vi "处理-输入数值.vi"(8 "error in (no error)":errorcluster caption="错误输入（无错误）", 11 "计算器类 输入":refnum<class "计算器类.lvclass">) -> (0 "error out":errorcluster caption="错误输出", 3 "计算器类 输出":refnum<class "计算器类.lvclass">)   [LabVIEW 2020, in "计算器类.lvclass"]
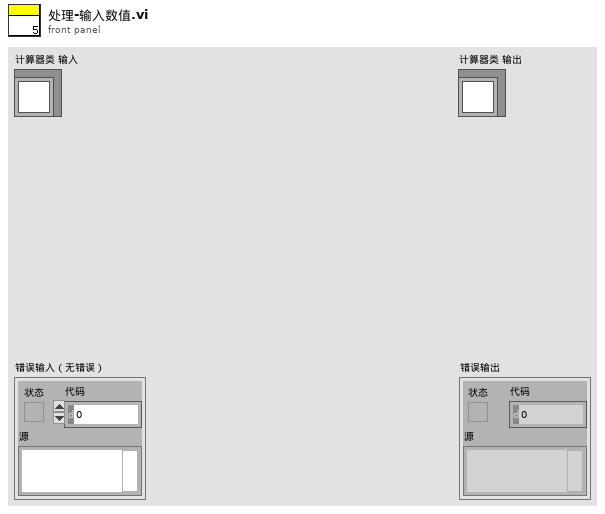
[diagram p1: front panel]
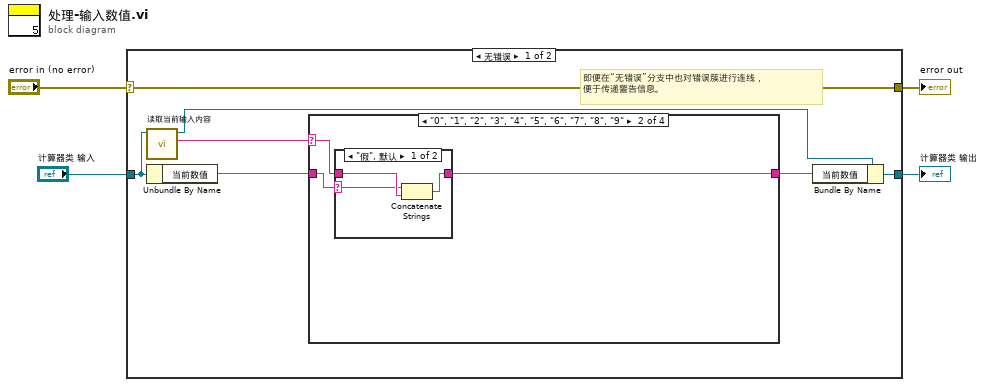
[diagram p0: block diagram]
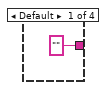
[diagram p2: hidden frame]
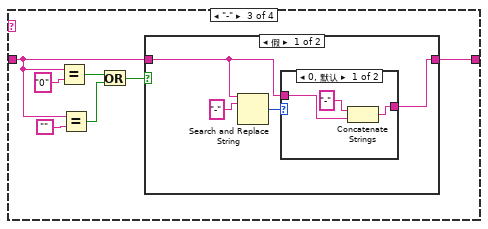
[diagram p4: hidden frame]
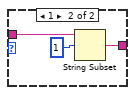
[diagram p5: hidden frame]
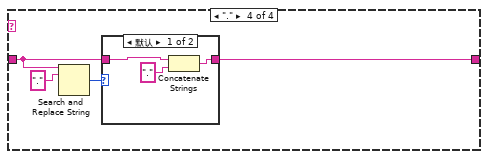
[diagram p7: hidden frame]
diagram:
  n1 = case shown="无错误" "error in (no error)" {
    selector: "error in (no error)" -> [w11 w47]
    tunnel: [w11 w47] -> w3
    tunnel: [w9 w46] -> w1
    tunnel: "计算器类 输入" -> [w6 w46]
    frame No Error {
      # "即便在“无错误”分支中也对错误簇进行连线，\n便于传递警告信息。"
      n2 = call "读取当前输入内容.vi"("计算器类输入"=w6) -> ("当前输入内容"=w7:string, "计算器类输出"=w5:refnum<class "计算器类.lvclass">)  [unwired: 8 in, 1 out]
      n3 = Unbundle By Name(w6) -> ("当前数值"=w10:string)
      n4 = case shown="\"0\", \"1\", \"2\", \"3\", \"4\", \"5\", \"6\", \"7\", \"8\", \"9\"" w7 {
        selector: w7 -> [_ w14 _ _]
        tunnel: w10 -> [_ w15 w21 w39]
        tunnel: ["" ("Value") w13 w20 w38] -> w8
        frame Default {
        }
        frame "0", "1", "2", "3", "4", "5", "6", "7", "8", "9" {
          n5 = case shown="\"假\", 默认" w15 {
            selector: w15 -> [w17 _]
            tunnel: w14 -> [w18 w19]
            tunnel: [w16 w19] -> w13
            frame "假", Default {
              n6 = Concatenate Strings(w17, w18) -> (w16:string)
            }
            frame "0" {
            }
          }
        }
        frame "-" {
          n7 = Equal?(x=w21, y="0") -> (x = y?=w24:bool)
          n8 = Equal?(x=w21, y="") -> (x = y?=w23:bool)
          n9 = Or(x=w24, y=w23) -> (x .or. y?=w22:bool)
          n10 = case shown="假" w22 {
            tunnel: w21 -> [w27 w37]
            tunnel: [w28 w37] -> w20
            frame False {
              n11 = Search and Replace String(input string=w27, search string="-") -> (number of replacements=w30:i32)  [unwired: 6 in, 3 out]
              n12 = case shown="0, 默认" w30 {
                tunnel: w27 -> [w32 w36]
                tunnel: [w31 w34] -> w28
                frame 0, Default {
                  n13 = Concatenate Strings("-", w32) -> (w31:string)
                }
                frame 1 {
                  n14 = String Subset(string=w36, offset (0)=1) -> (substring=w34:string)  [unwired: 1 in]
                }
              }
            }
            frame True {
            }
          }
        }
        frame "." {
          n15 = Search and Replace String(input string=w39, search string=".") -> (number of replacements=w40:i32)  [unwired: 6 in, 3 out]
          n16 = case shown="默认" w40 {
            tunnel: w39 -> [w44 w45]
            tunnel: [w42 w45] -> w38
            frame Default {
              n17 = Concatenate Strings(w44, ".") -> (w42:string)
            }
            frame 1 {
            }
          }
        }
      }
      n18 = Bundle By Name(cluster=w5, "当前数值"=w8) -> (w9:refnum<class "计算器类.lvclass">)
    }
    frame Error {
    }
  }
  "error out" <- w3
  "计算器类 输出" <- w1
